vi "OCR_sudoku_solver.vi"() -> ()   [LabVIEW 2020]
panel:
  out "1-bit pixmap":bool[][](array[boolean])
  out "BW cell":picture
  in  "subset rect":T1
  out "BW picture":picture
  in  "Jpeg path":path
  # "OCR Sudoku solver"
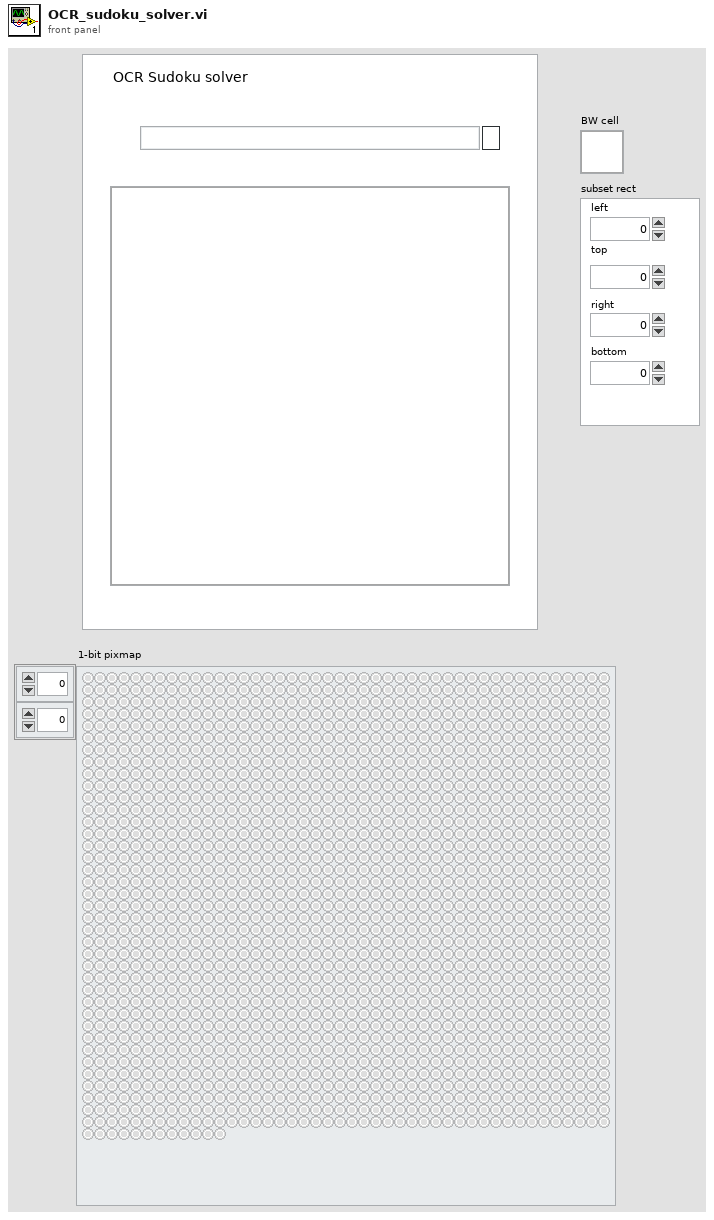
[diagram p1: front panel]
types:
  T1 = cluster{"left":i16, "top":i16, "right":i16, "bottom":i16}
  T2 = typedef "imagedata.ctl" = cluster{"image type":i32, "image depth":i32, "image":u8[], "mask":u8[], "colors":u32[], "Rectangle":cluster{"left":i16, "top":i16, "right":i16, "bottom":i16}}
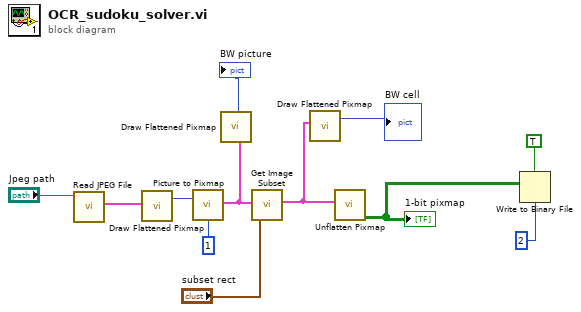
[diagram p0: block diagram]
diagram:
  n1 = call <vilib>:"Read JPEG File.vi"("path to JPEG file"="Jpeg path") -> ("image data"=w11:T2)  [unwired: 8 in, 2 out]
  n2 = call <vilib>:"Draw Flattened Pixmap.vi"("image data"=w11) -> ("new picture"=w10:picture)  [unwired: 8 in]
  n3 = call <vilib>:"Picture to Pixmap.vi"("depth"=1, "picture"=w10) -> ("image data"=w8:T2)  [unwired: 8 in, 1 out]
  n4 = call <vilib>:"Draw Flattened Pixmap.vi"("image data"=w8) -> ("new picture"=→"BW picture":picture)  [unwired: 8 in]
  n5 = call <vilib>:"Get Image Subset.vi"("subset rect"="subset rect", "image data"=w8) -> ("image subset"=w4:T2)  [unwired: 4 in, 1 out]
  n6 = call <vilib>:"Draw Flattened Pixmap.vi"("image data"=w4) -> ("new picture"=→"BW cell":picture)  [unwired: 8 in]
  n7 = call <vilib>:"Unflatten Pixmap.vi"("image data"=w4) -> ("1-bit pixmap"=w3:bool[][])  [unwired: 4 in, 6 out]
  "1-bit pixmap" <- w3
  n8 = Write to Binary File(data=w3, 5:TRUE, 9:2) -> ()  [unwired: 3 in, 3 out]
